vi "CS++DebugDevices-Content.vi"() -> (0 "CS++Classes & Messages":T1(array[cluster]))   [LabVIEW 2015]
doc: "Place actor and class constants that should be included included in an application on the blockdiagramm."
uses:
  CSPP_Core/Actors/CS++BaseActor/CS++BaseActor.lvclass
  CSPP_SimMotor/CS++SimMotor.lvclass
  CSPP_TestMotor/CS++TestMotor.lvclass
  <vilib>/ActorFramework/Message/Message.lvclass
panel:
  # "Place actor and class constants on the blockdiagramm."
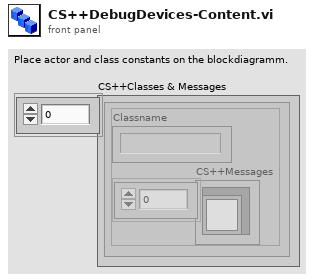
[diagram p1: front panel]
types:
  T1 = cluster{"Classname":string, "CS++Messages":refnum<class "Message.lvclass">[]}[]
  T2 = cluster{"class name":string, "CS++Messages":refnum<class "Message.lvclass">[]}
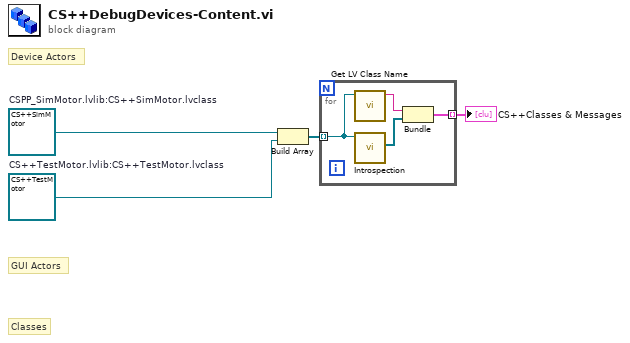
[diagram p0: block diagram]
diagram:
  w1 = refnum<class "CS++TestMotor.lvclass"> refnum  # CS++TestMotor.lvlib:CS++TestMotor.lvclass
  w3 = refnum<class "CS++SimMotor.lvclass"> refnum  # CSPP_SimMotor.lvlib:CS++SimMotor.lvclass
  # "Classes"
  # "GUI Actors"
  # "Device Actors"
  n1 = Build Array(w3, w1) -> (w2:refnum<class>[])
  n2 = for {
    tunnel: w2 -> [w8] mode=indexing
    tunnel: [w5] -> w4 mode=indexing
    n3 = call <vilib>:"Get LV Class Name.vi"("object"=w8) -> ("class name"=w7:string)  [unwired: 9 in, 1 out]
    n4 = call "Introspection.vi"("CS++BaseActor in"=w8) -> ("CS++Messages"=w6:refnum<class "Message.lvclass">[])  [unwired: 8 in, 2 out]
    n5 = Bundle("class name"=w7, "CS++Messages"=w6) -> (w5:T2)  [unwired: 1 in]
  }
  "CS++Classes & Messages" <- w4
